vi "DAQmx Create Channel (CO-Pulse Generation-Frequency).vi"(0 "task in":refnum<k21>, 1 "frequency":dbl=1.0 format="%.6f", 2 "duty cycle":dbl=0.5 format="%.6f", 5 "counter":tag, 7 "name to assign":string, 9 "units":i32(ring)=10373 items=["Hz"=10373], 11 "error in":errorcluster, 12 "idle state":i32(ring)=10214 items=["High"=10192, "Low"=10214], 13 "initial delay":dbl format="%.6f") -> (4 "task out":refnum<k21>, 15 "error out":errorcluster)   [LabVIEW 2020]
doc: "Creates channel(s) to generate digital pulses that <B>frequency</B> and <B>duty cycle</B> define. The pulses appear on the default output terminal of the counter unless you select a different output terminal."
uses:
  nilvaiu.dll
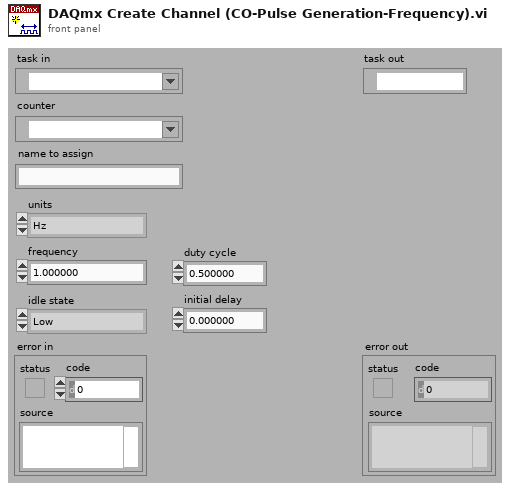
[diagram p1: front panel]
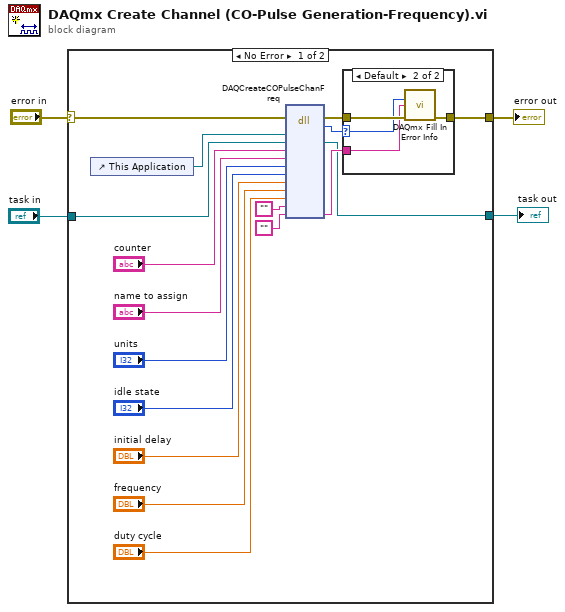
[diagram p0: block diagram]
diagram:
  n1 = case shown="No Error" "error in" {
    selector: "error in" -> [w6 w28]
    tunnel: "task in" -> [w9 w27]
    tunnel: [w8 w27] -> w3
    tunnel: [w7 w28] -> w2
    frame No Error {
      n2 = control-ref of="This Application"() -> (w18:refnum<vi>)
      n3 = dll-call lib="nilvaiu.*" fn="DAQCreateCOPulseChanFreq"(error in=w6, "lvAppRef"=w18, "refObjPtr"=w9, "counter"="counter", "channelNameIn"="name to assign", "units"="units", "idleState"="idle state", "initialDelay"="initial delay", "freq"="frequency", "dutyCycle"="duty cycle", "channelNamesOut"="", "extendedErrorInfo"="") -> (error out=w21:errorcluster, "return type"=w20:i32, "refObjPtr"=w8:refnum<k21>, "extendedErrorInfo"=w19:string)  [unwired: 11 in, 1 out]
      n4 = case shown="Default" w20 {
        selector: w20 -> [_ w24]
        tunnel: w21 -> [w22 w26]
        tunnel: [w22 w25] -> w7
        tunnel: w19 -> [_ w23]
        frame 0 {
        }
        frame Default {
          n5 = call "DAQmx Fill In Error Info.vi"("status code"=w24, "extended error info"=w23, "error in"=w26) -> ("error out"=w25:errorcluster)  [unwired: 1 in, 11 out]
        }
      }
    }
    frame Error {
    }
  }
  "error out" <- w2
  "task out" <- w3
